vi "niDTS BT UTIL CH to Freq.vi"(8 "error in (no error)":errorcluster, 10 "BT Standard":T1 caption="802.11 Standard", 11 "Channel":i32) -> (0 "error out":errorcluster, 3 "Frequency":dbl=2402000000.0)   [LabVIEW 2015, in "niDTS BT.lvlib"]
uses:
  niDTS BT.lvlib
  Includes/niDTS BT INC Standard.ctl
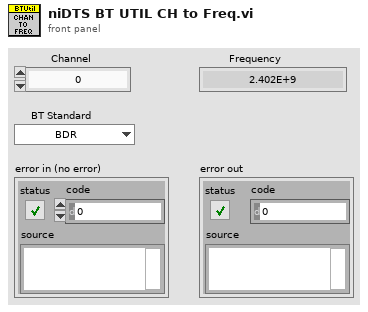
[diagram p1: front panel]
types:
  T1 = typedef "niDTS BT.lvlib/niDTS BT INC Standard.ctl" = enum16{"BDR", "EDR", "LE-TP"}
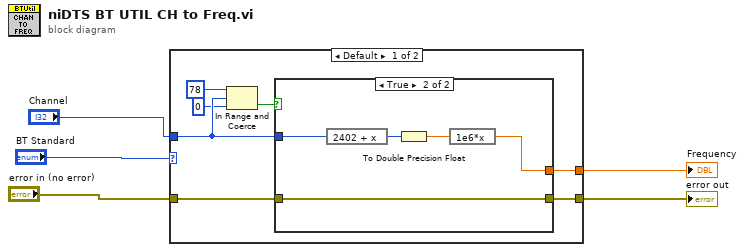
[diagram p0: block diagram]
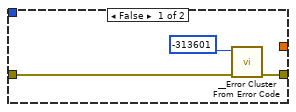
[diagram p2: hidden frame]
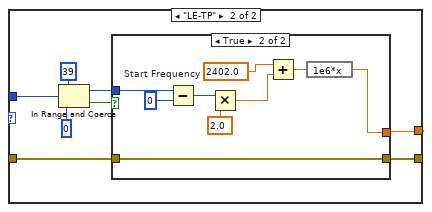
[diagram p3: hidden frame]
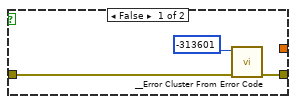
[diagram p4: hidden frame]
diagram:
  n1 = case shown="Default" "BT Standard" {
    tunnel: "Channel" -> [w11 w25]
    tunnel: [w10 w24] -> w3
    tunnel: "error in (no error)" -> [w9 w22]
    tunnel: [w8 w21] -> w4
    frame Default {
      n2 = In Range and Coerce(upper limit=u16 78 ("lower limit"), x=w11, lower limit=u16 0 ("upper limit")) -> (In Range?=w12:bool)  [unwired: 1 out]
      n3 = case shown="True" w12 {
        tunnel: w11 -> [_ w17]
        tunnel: [_ w16] -> w10
        tunnel: w9 -> [w14 w20]
        tunnel: [w13 w20] -> w8
        frame False {
          n4 = call "__Error Cluster From Error Code.vi"("error in (no error)"=w14, "error code (0)"=-313601) -> ("error out"=w13:errorcluster)  [unwired: 7 in]
        }
        frame True {
          n5 = expression code="2402 + x"(w17) -> (w19:i32)
          n6 = To Double Precision Float(number=w19) -> (double precision float=w18:dbl)
          n7 = expression code="1e6*x"(w18) -> (w16:dbl)
        }
      }
    }
    frame "LE-TP" {
      n8 = In Range and Coerce(upper limit=39 ("y"), x=w25, lower limit=0 ("y")) -> (coerced(x)=w27:i32, In Range?=w23:bool)
      n9 = case shown="True" w23 {
        tunnel: w27 -> [_ w37]
        tunnel: [_ w34] -> w24
        tunnel: w22 -> [w30 w32]
        tunnel: [w29 w32] -> w21
        frame False {
          n10 = call "__Error Cluster From Error Code.vi"("error in (no error)"=w30, "error code (0)"=-313601) -> ("error out"=w29:errorcluster)  [unwired: 7 in]
        }
        frame True {
          w35 = 2402.0  # Start Frequency
          n11 = Subtract(x=w37, y=0) -> (x-y=w36:i32)
          n12 = Multiply(x=w36, y=2.0) -> (x*y=w39:dbl)
          n13 = Add(x=w35, y=w39) -> (x+y=w40:dbl)
          n14 = expression code="1e6*x"(w40) -> (w34:dbl)
        }
      }
    }
  }
  "error out" <- w4
  "Frequency" <- w3
